vi "Clean-up.vi"(8 "error in (no error)":errorcluster, 11 "File in":refnum<class "File.lvclass">) -> (0 "error out":errorcluster, 3 "File out":refnum<class "File.lvclass">)   [LabVIEW 2016, in "File.lvclass"]
uses:
  File.lvclass
  File.lvclass/File.ctl
  Write tdms stream.vi
  Read Is open.vi
  Read tdms stream.vi
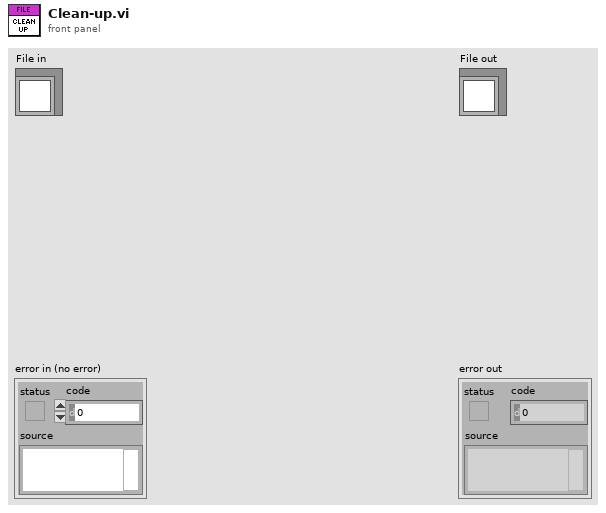
[diagram p1: front panel]
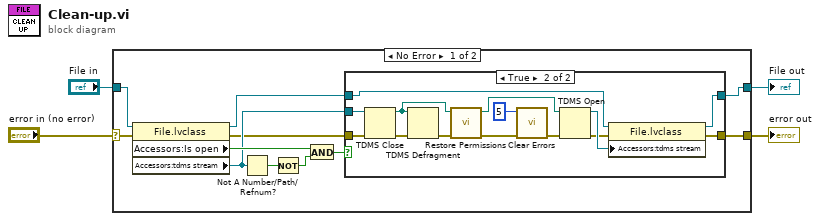
[diagram p0: block diagram]
diagram:
  n1 = case shown="No Error" "error in (no error)" {
    selector: "error in (no error)" -> [w6 w33]
    tunnel: [w5 w33] -> w3
    tunnel: [w7 w32] -> w1
    tunnel: "File in" -> [w12 w32]
    frame No Error {
      n2 = property class="File.lvclass"(reference=w12, error in=w6) -> (reference out=w8:refnum<class "File.lvclass">, error out=w10:errorcluster, "Accessors:Is open"=w13:bool, "Accessors:tdms stream"=w11:refnum<k34>)
      n3 = Not A Number/Path/Refnum?(number/path/refnum=w11) -> (NaN/Path/Refnum?=w14:bool)
      n4 = Not(x=w14) -> (.not. x?=w15:bool)
      n5 = And(x=w13, y=w15) -> (x .and. y?=w9:bool)
      n6 = case shown="True" w9 {
        tunnel: w11 -> [_ w31]
        tunnel: w10 -> [w17 w30]
        tunnel: w8 -> [w16 w27]
        tunnel: [w16 w24] -> w7
        tunnel: [w17 w23] -> w5
        frame False {
        }
        frame True {
          n7 = TDMS Close(8:w30, 11:w31) -> (0:w29:errorcluster, 3:w18:path)
          n8 = TDMS Defragment(4:w29, 7:w18) -> (0:w28:errorcluster)
          n9 = call "Restore Permissions.vi"("Error In"=w28, "File Path"=w18) -> ("Error Out"=w20:errorcluster, "Duplicate File Path"=w19:path)  [unwired: 6 in, 2 out]
          n10 = call <vilib>:"Clear Errors.vi"("error in (no error)"=w20, "specific error code to clear (0: all)"=5) -> ("error out"=w22:errorcluster)  [unwired: 4 in, 1 out]
          n11 = TDMS Open(8:w22, 11:w19) -> (0:w25:errorcluster, 3:w26:refnum<k34>)  [unwired: 5 in]
          n12 = property class="File.lvclass"(reference=w27, error in=w25, "Accessors:tdms stream"=w26) -> (reference out=w24:refnum<class "File.lvclass">, error out=w23:errorcluster)
        }
      }
    }
    frame Error {
    }
  }
  "error out" <- w3
  "File out" <- w1
